vi "Area and Validity of a Triangle.vi"() -> ()   [LabVIEW 2012]
panel:
  out "三角形面积":dbl
  out "有效三角形？":bool
  in  "C边(cm)":dbl=10.0
  in  "B边(cm)":dbl=8.0
  in  "A边(cm)":dbl=6.0
  # "三角形的边"
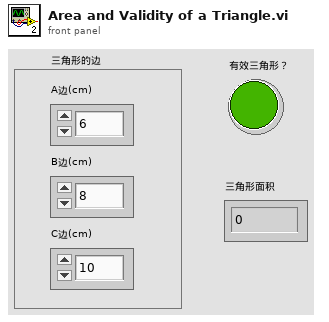
[diagram p1: front panel]
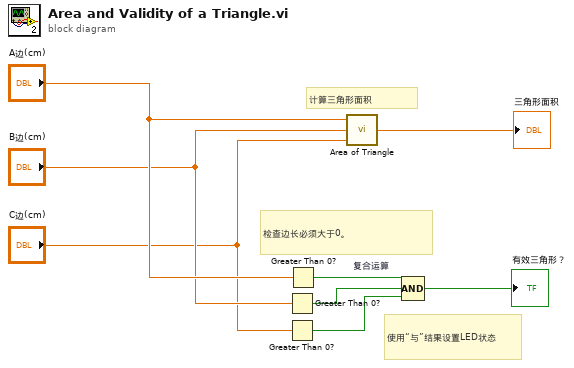
[diagram p0: block diagram]
diagram:
  # "使用“与”结果设置LED状态"
  # "检查边长必须大于0。"
  # "计算三角形面积"
  n1 = Greater Than 0? ("大于0？")(x="B边(cm)") -> (x > 0?=w6:bool)
  n2 = Greater Than 0? ("大于0？")(x="C边(cm)") -> (x > 0?=w5:bool)
  n3 = Greater Than 0? ("大于0？")(x="A边(cm)") -> (x > 0?=w7:bool)
  n4 = call "Area of Triangle.vi"("C边(cm)"="C边(cm)", "B边(cm)"="B边(cm)", "A边(cm)"="A边(cm)") -> ("三角形面积(cm^2)"=→"三角形面积":dbl)
  n5 = Compound Arithmetic op=AND "复合运算"(w7, w6, w5) -> (→"有效三角形？":bool)
